vi "ReverseDrive.vi"(1 "InitLeft":dbl, 2 "InitRight":dbl) -> (8 "Final Left":dbl, 9 "FinalRight":dbl)   [LabVIEW 2013]
uses:
  State_Machine_Enum.ctl
  Sally_Dashboard_2014/DBNameEnum.ctl
  Robot Global Data.vi
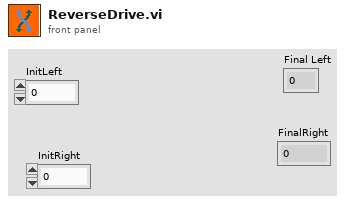
[diagram p1: front panel]
types:
  T1 = typedef "State_Machine_Enum.ctl" = enum16{"Idle", "Start", "Do", "Stop", "Init"}
  T2 = typedef "DBNameEnum.ctl" = enum16{"AutoInstructions", "DriveLoopTime", "DriveAlignLSLeft", "DriveAlignLSRight", "Use2DriveAlign", "ClimbLS", "LauncherAngleMatches", "FrameworkVersion", "sLauncherAngle", "LauncherTargetAngle", "sLauncherRPM", "LauncherTargetRPM", "sDriveDistance", "LauncherMotorValue", "PullbackTol", "FireTol", "LauncherRPMTol", "LauncherAngleTol", "InitialWait", "WaitBetweenLaunch", "AnglePresets", "RPMPresets", "UseAngleEncoder", "UseLauncherEncoder", "UseLauncherPID", "QSWaitBeforeFire", "QSWaitBeforeRetract", "AngleForwardValue", "AngleBackwardValue", "UseClusterArray", "BackupAuto", "ReverseDriveIndicate", "HalfSpeedFactor"}
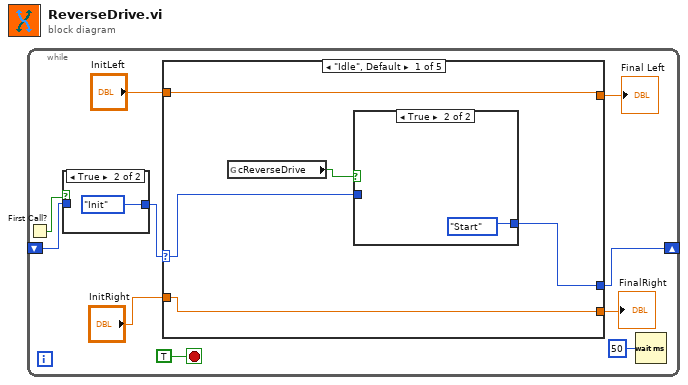
[diagram p0: block diagram]
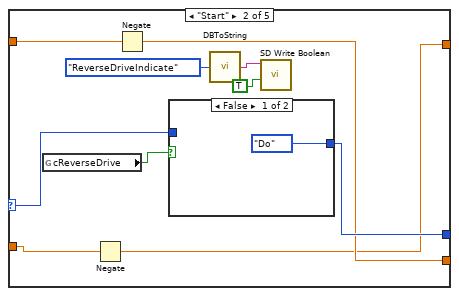
[diagram p4: hidden frame]
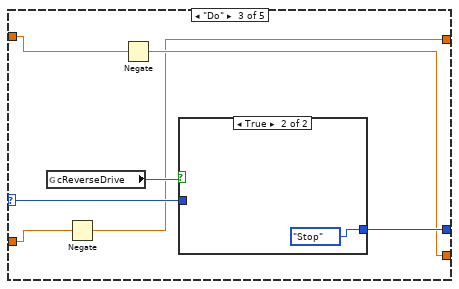
[diagram p6: hidden frame]
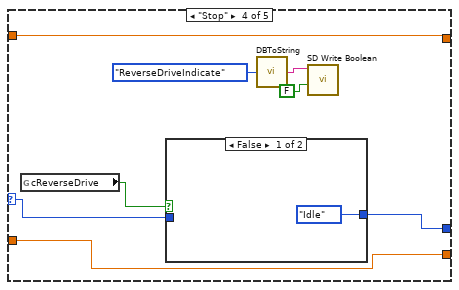
[diagram p8: hidden frame]
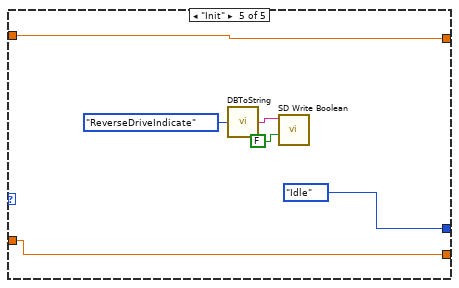
[diagram p10: hidden frame]
diagram:
  n1 = while {
    shift-right: [w9] -> _
    shift-left: _ -> [w1]
    stop <- TRUE stop-if-true
    n2 = First Call?() -> (First Call?: T/F=w3:bool)
    n3 = case shown="True" w3 {
      tunnel: [w11 State_Machine_Enum."Init" ("State")] -> w2
      tunnel: w1 -> [w11 _]
      frame False {
      }
      frame True {
      }
    }
    n4 = case shown="\"Idle\", Default" w2 {
      selector: w2 -> [w16 w28 w37 w47 _]
      tunnel: [w17 w29 w38 w48 State_Machine_Enum."Idle" ("State")] -> w9
      tunnel: "InitLeft" -> [w14 w26 w35 w44 w55]
      tunnel: "InitRight" -> [w13 w24 w33 w45 w54]
      tunnel: [w14 w23 w32 w44 w55] -> w5
      tunnel: [w13 w25 w34 w45 w54] -> w4
      frame "Idle", Default {
        n5 = global read "Robot Global Data.vi" "cReverseDrive"() -> (w15:bool)
        n6 = case shown="True" w15 {
          tunnel: [w18 State_Machine_Enum."Start" ("State")] -> w17
          tunnel: w16 -> [w18 _]
          frame False {
          }
          frame True {
          }
        }
      }
      frame "Start" {
        n7 = global read "Robot Global Data.vi" "cReverseDrive"() -> (w27:bool)
        n8 = Negate(x=w24) -> (-x=w23:dbl)
        n9 = Negate(x=w26) -> (-x=w25:dbl)
        n10 = case shown="False" w27 {
          tunnel: [State_Machine_Enum."Do" ("State") w31] -> w29
          tunnel: w28 -> [_ w31]
          frame False {
          }
          frame True {
          }
        }
        n11 = call "DBToString.vi"("Enum"=DBNameEnum."ReverseDriveIndicate") -> ("Refname"=w20:string)
        n12 = call <vilib>:"SD Write Boolean.vi"("Boolean"=TRUE, "Name"=w20) -> ()  [unwired: 8 in, 2 out]
      }
      frame "Do" {
        n13 = global read "Robot Global Data.vi" "cReverseDrive"() -> (w36:bool)
        n14 = Negate(x=w33) -> (-x=w32:dbl)
        n15 = Negate(x=w35) -> (-x=w34:dbl)
        n16 = case shown="True" w36 {
          tunnel: [w39 State_Machine_Enum."Stop" ("State")] -> w38
          tunnel: w37 -> [w39 _]
          frame False {
          }
          frame True {
          }
        }
      }
      frame "Stop" {
        n17 = global read "Robot Global Data.vi" "cReverseDrive"() -> (w46:bool)
        n18 = case shown="False" w46 {
          tunnel: [State_Machine_Enum."Idle" ("State") w50] -> w48
          tunnel: w47 -> [_ w50]
          frame False {
          }
          frame True {
          }
        }
        n19 = call "DBToString.vi"("Enum"=DBNameEnum."ReverseDriveIndicate") -> ("Refname"=w41:string)
        n20 = call <vilib>:"SD Write Boolean.vi"("Boolean"=FALSE, "Name"=w41) -> ()  [unwired: 8 in, 2 out]
      }
      frame "Init" {
        n21 = call "DBToString.vi"("Enum"=DBNameEnum."ReverseDriveIndicate") -> ("Refname"=w51:string)
        n22 = call <vilib>:"SD Write Boolean.vi"("Boolean"=FALSE, "Name"=w51) -> ()  [unwired: 8 in, 2 out]
      }
    }
    "FinalRight" <- w4
    "Final Left" <- w5
    n23 = Wait (ms)(milliseconds to wait=u32 50) -> ()  [unwired: 1 out]
  }
